vi "CalculationsRelXRelYMouseAngle_171213.vi"(0 "sina":sgl, 1 "R from center":sgl, 2 "MouseXc":sgl, 3 "Mouse Yc":sgl, 4 "x1-x2":sgl, 5 "y1-y2":sgl) -> (13 "Mouse angle":sgl, 14 "phi":sgl, 15 "Rel X":sgl, 16 "Rel Y":sgl, 17 "from center towards mouse":sgl, 18 "Cage rotation":sgl, 19 "mouse wall angle":sgl)   [LabVIEW 2016]
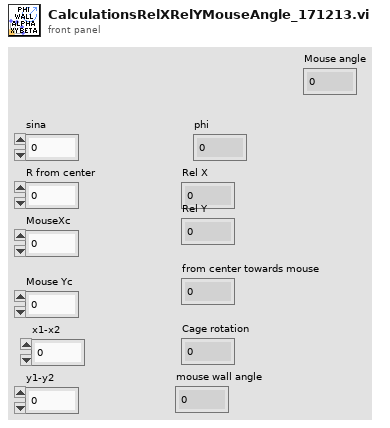
[diagram p1: front panel]
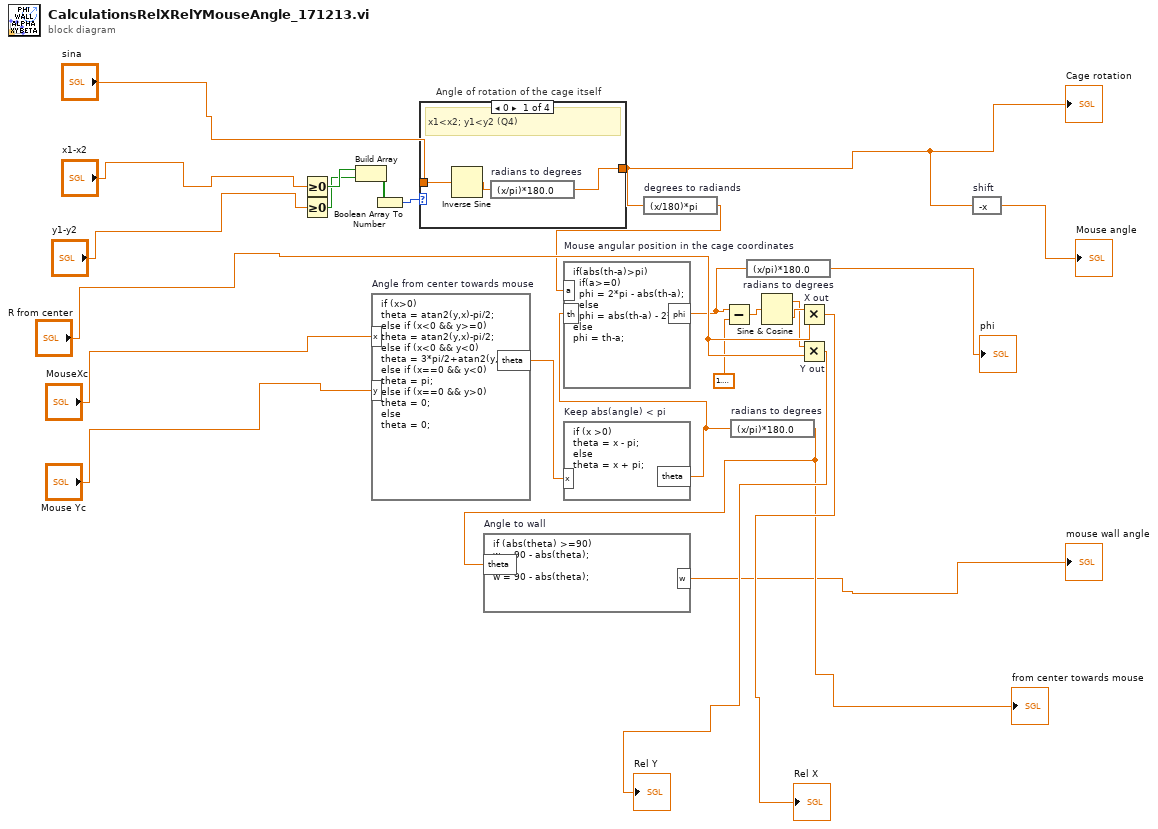
[diagram p0: block diagram]
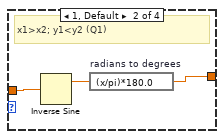
[diagram p2: hidden frame]
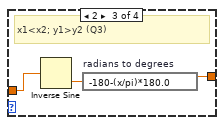
[diagram p3: hidden frame]
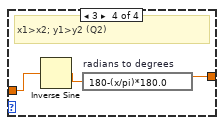
[diagram p4: hidden frame]
diagram:
  n1 = Greater Or Equal To 0?(x="x1-x2") -> (x >= 0?=w14:bool)
  n2 = Greater Or Equal To 0?(x="y1-y2") -> (x >= 0?=w13:bool)
  n3 = Build Array(w14, w13) -> (w12:bool[])
  n4 = formula code="if (x>0)\ntheta = atan2(y,x)-pi/2;\nelse if (x<0 && y>=0)\ntheta = atan2(y,x)-pi/2;\nelse if (x<0 && y<0)\ntheta = 3*pi/2+atan2(y,x);\nelse if (x==0 && y<0)\ntheta = pi;\nelse if (x==0 && y>0)\ntheta = 0;\nelse\ntheta = 0;" "Angle from center towards mouse"("x"="MouseXc", "y"="Mouse Yc") -> ("theta"=w10:dbl)
  n5 = Boolean Array To Number(Boolean array=w12) -> (number=w11:u32)
  n6 = case "Angle of rotation of the cage itself" shown="0" w11 {
    tunnel: "sina" -> [w27 w30 w33 w36]
    tunnel: [w26 w29 w32 w35] -> w2
    frame 0 {
      # "x1<x2; y1<y2 (Q4)"
      n7 = Inverse Sine(1:w27) -> (0:w28:sgl)
      n8 = expression code="(x/pi)*180.0" "radians to degrees"(w28) -> (w26:sgl)
    }
    frame 1, Default {
      # "x1>x2; y1<y2 (Q1)"
      n9 = Inverse Sine(1:w30) -> (0:w31:sgl)
      n10 = expression code="(x/pi)*180.0" "radians to degrees"(w31) -> (w29:sgl)
    }
    frame 2 {
      # "x1<x2; y1>y2 (Q3)"
      n11 = Inverse Sine(1:w33) -> (0:w34:sgl)
      n12 = expression code="-180-(x/pi)*180.0" "radians to degrees"(w34) -> (w32:sgl)
    }
    frame 3 {
      # "x1>x2; y1>y2 (Q2)"
      n13 = Inverse Sine(1:w36) -> (0:w37:sgl)
      n14 = expression code="180-(x/pi)*180.0" "radians to degrees"(w37) -> (w35:sgl)
    }
  }
  "Cage rotation" <- w2
  n15 = formula code="if (x >0)\ntheta = x - pi;\nelse\ntheta = x + pi;" "Keep abs(angle) < pi"("x"=w10) -> ("theta"=w7:dbl)
  n16 = expression code="(x/180)*pi" "degrees to radiands"(w2) -> (w6:sgl)
  n17 = formula code="if(abs(th-a)>pi)\n  if(a>=0)\n  phi = 2*pi - abs(th-a);\n  else\n  phi = abs(th-a) - 2*pi;\nelse\nphi = th-a;" "Mouse angular position in the cage coordinates"("th"=w7, "a"=w6) -> ("phi"=w4:dbl)
  n18 = Subtract(x=w4, y=1.5707963267948966) -> (x-y=w5:dbl)
  n19 = expression code="(x/pi)*180.0" "radians to degrees"(w7) -> (w23:dbl)
  "from center towards mouse" <- w23
  n20 = formula code="if (abs(theta) >=90)\nw = 90 - abs(theta);\nelse\nw = 90 - abs(theta);" "Angle to wall"("theta"=w23) -> ("w"=→"mouse wall angle":dbl)
  n21 = expression code="(x/pi)*180.0" "radians to degrees"(w4) -> (→"phi":dbl)
  n22 = Sine & Cosine(0:w5) -> (1:w8:dbl, 2:w9:dbl)
  n23 = Multiply "X out"(x=w9, y="R from center") -> (x*y=→"Rel X":dbl)
  n24 = Multiply "Y out"(x=w8, y="R from center") -> (x*y=→"Rel Y":dbl)
  n25 = expression code="-x" "shift"(w2) -> (→"Mouse angle":sgl)
